vi "Make from Test Case Path.vi"(8 "error in (no error)":errorcluster, 10 "Test Case":path) -> (0 "error out":errorcluster, 3 "LUnit Test Suite Out":refnum<class "LUnit Test Suite.lvclass">)   [LabVIEW 2020, in "LUnit Test Suite.lvclass"]
uses:
  LUnit Test Suite.lvclass
  LUnit Test Case/LUnit Test Case.lvclass/LUnit Test Case.ctl
  LUnit Test Case/LUnit Test Case.lvclass
  C:/git/astemes-lunit/source/Core/Runnable/Runnable.lvclass
  <vilib>/Utility/LVClass/Get LV Class Default Value.vi
  <vilib>/Utility/LVClass/Get LV Class Name.vi
  LUnit Test Suite.lvclass/LUnit Test Suite.ctl
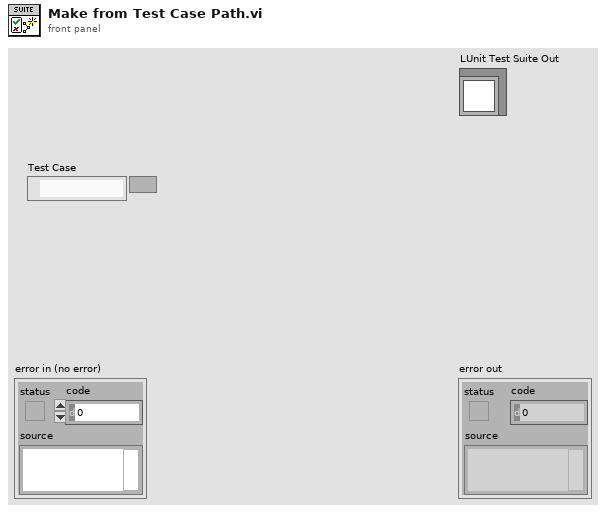
[diagram p1: front panel]
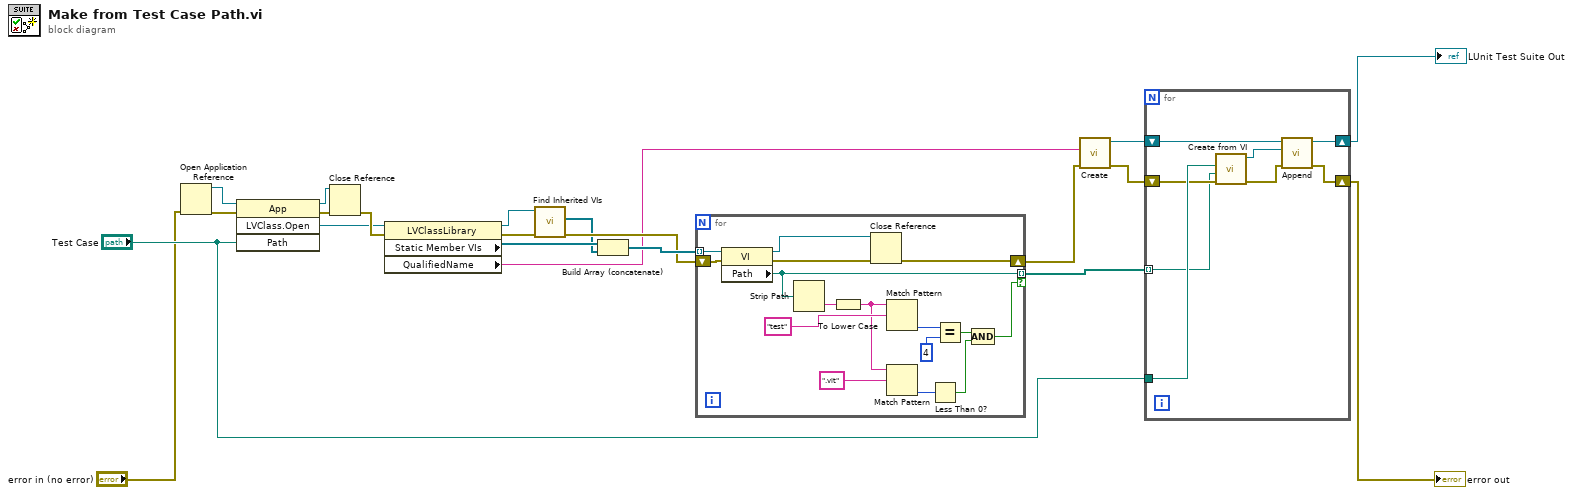
[diagram p0: block diagram]
diagram:
  n1 = Open Application Reference(8:"error in (no error)") -> (0:w19:errorcluster, 3:w20:refnum<vi>)  [unwired: 3 in]
  n2 = invoke class="App" method="LVClass.Open"(reference=w20, error in=w19, "Path"="Test Case") -> (reference out=w14:refnum<vi>, error out=w18:errorcluster, "LVClass.Open"=w11:refnum<vi>)  [unwired: 1 in, 1 out]
  n3 = Close Reference(reference=w14, error in (no error)=w18) -> (error out=w15:errorcluster)
  n4 = property class="LVClassLibrary"(reference=w11, error in=w15) -> (reference out=w1:refnum<vi>, error out=w2:errorcluster, "Static Member VIs"=w17:refnum<vi>[], "QualifiedName"=w3:string)
  n5 = call "Find Inherited VIs.vi"("error in (no error)"=w2, "LVClassLibrary in"=w1) -> ("error out"=w10:errorcluster, "Inherited Dynamic Member VIs"=w9:refnum<vi>[])  [unwired: 8 in]
  n6 = Build Array (concatenate)(w17, w9) -> (w13:refnum<vi>[])
  n7 = for {
    tunnel: w13 -> [w37] mode=indexing
    tunnel: [w28] -> w16 mode=indexing if=w23
    shift-right: [w30] -> w4
    shift-left: w10 -> [w32]
    n8 = property class="VI"(reference=w37, error in=w32) -> (reference out=w29:refnum<vi>, error out=w31:errorcluster, "Path"=w28:path)
    n9 = Strip Path(path=w28) -> (name=w27:string)  [unwired: 1 out]
    n10 = To Lower Case(string=w27) -> (all lower case string=w26:string)
    n11 = Close Reference(reference=w29, error in (no error)=w31) -> (error out=w30:errorcluster)
    n12 = Match Pattern(string=w26, regular expression="test") -> (offset past match=w35:i32)  [unwired: 1 in, 3 out]
    n13 = Match Pattern(string=w26, regular expression=".vit") -> (offset past match=w24:i32)  [unwired: 1 in, 3 out]
    n14 = Less Than 0?(x=w24) -> (x < 0?=w22:bool)
    n15 = Equal?(x=w35, y=4) -> (x = y?=w33:bool)
    n16 = Compound Arithmetic op=AND(w33, w22) -> (w23:bool)
  }
  n17 = call "Create.vi"("error in (no error)"=w4, "Suite Name"=w3) -> ("error out"=w5:errorcluster, "LUnit Test Suite Out"=w8:refnum<class "LUnit Test Suite.lvclass">)  [unwired: 8 in]
  n18 = for {
    tunnel: "Test Case" -> [w45]
    tunnel: w16 -> [w39] mode=indexing
    shift-right: [w43] -> w7
    shift-left: w8 -> [w44]
    shift-right: [w41] -> w6
    shift-left: w5 -> [w40]
    n19 = call "Create from VI.vi"("error in (no error)"=w40, "Test Method VI Path"=w39, "Test Case LVCLass Path"=w45) -> ("error out"=w42:errorcluster, "LUnit Test Case Out"=w38:refnum<class "LUnit Test Case.lvclass">)  [unwired: 7 in]
    n20 = call "Append.vi"("error in (no error)"=w42, "Runnable"=w38, "LUnit Test Suite In"=w44) -> ("error out"=w41:errorcluster, "LUnit Test Suite Out"=w43:refnum<class "LUnit Test Suite.lvclass">)  [unwired: 7 in]
  }
  "error out" <- w6
  "LUnit Test Suite Out" <- w7
